vi "Get Color.vi"(8 "error in (no error)":errorcluster, 11 "Geometric Object.lvclass in":refnum<class "Graphics Object.lvclass">) -> (0 "error out":errorcluster, 2 "Color.lvclass":refnum<class "Color.lvclass">, 3 "Geometric Object.lvclass out":refnum<class "Graphics Object.lvclass">)   [LabVIEW 2018, in "Graphics Object.lvclass"]
doc: "A method for getting the color of a graphics objects"
uses:
  Graphics Object.lvclass
  Color/Color.lvclass
  Graphics Object.lvclass/Graphics Object.ctl
panel:
  # "expressionflow.com"
  # "Copyright (c) 2008 Tomi Maila. All rights reserved."
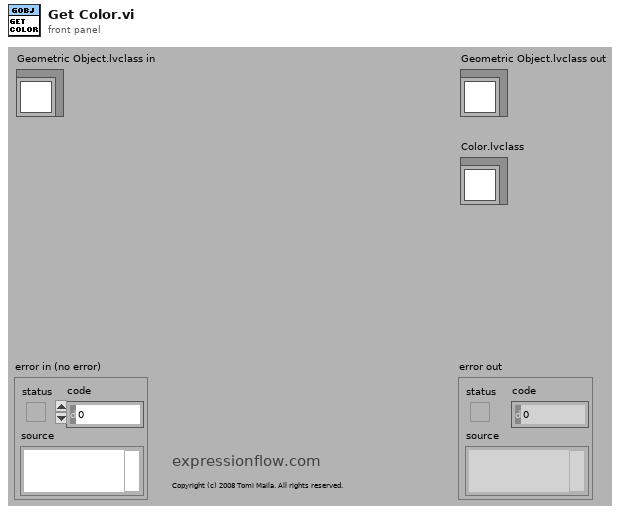
[diagram p1: front panel]
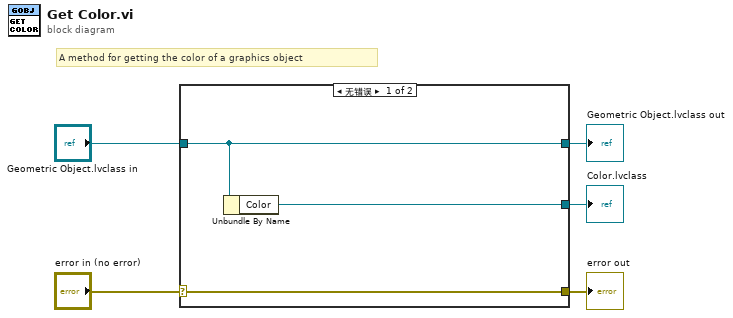
[diagram p0: block diagram]
diagram:
  # "A method for getting the color of a graphics object"
  n1 = case shown="无错误" "error in (no error)" {
    selector: "error in (no error)" -> [w8 w9]
    tunnel: [w8 w9] -> w4
    tunnel: [w7 w10] -> w2
    tunnel: "Geometric Object.lvclass in" -> [w7 w10]
    tunnel: [w6 _] -> w1
    frame No Error {
      n2 = Unbundle By Name(w7) -> ("Color"=w6:refnum<class "Color.lvclass">)
    }
    frame Error {
    }
  }
  "error out" <- w4
  "Geometric Object.lvclass out" <- w2
  "Color.lvclass" <- w1
